vi "Parse updateConnectionState.vi"(8 "error in (no error)":errorcluster, 11 "JSON (UTF-8) String":string) -> (0 "error out":errorcluster, 2 "Telegram State":T1)   [LabVIEW 2015, in "JSON Library.lvlib"]
doc: "Created IvanLis by LabVIEW Portal\nProfile: http://labviewportal.org/memberlist.php?mode=viewprofile&u=987\neMail: IvanLisanov@gMail.com\nTelegram: https://t.me/IvanLis"
uses:
  JSON Library.lvlib
  Telegram Library/TypeDef/Telegram State.ctl
  Telegram Library/Telegram Library.lvlib
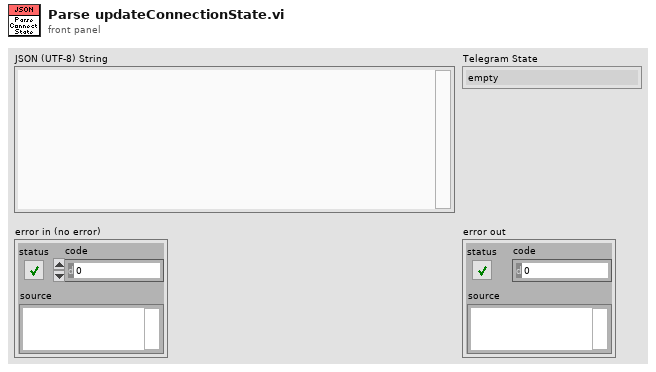
[diagram p1: front panel]
types:
  T1 = typedef "Telegram Library.lvlib/Telegram State.ctl" = enum16{"empty", "ok", "authorizationStateClosed", "authorizationStateWaitTdlibParameters", "authorizationStateWaitEncryptionKey", "authorizationStateWaitPhoneNumber", "authorizationStateWaitCode", "connectionStateWaitingForNetwork", "connectionStateConnectingToProxy", "connectionStateUpdating", "connectionStateConnecting", "connectionStateReady", "updateUser_user", "updateNewChat_chat", "updateNewMessage_Text", "updateChatLastMessage_Text", "updateDeleteMessages", "updateChatPosition", "ChatHistoryMessages_Text"}
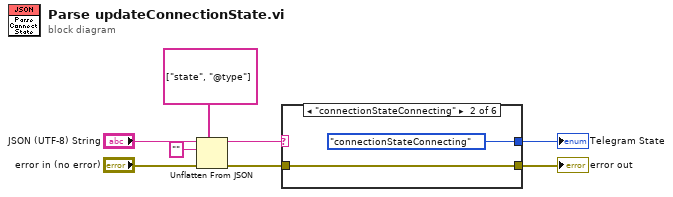
[diagram p0: block diagram]
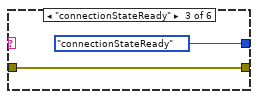
[diagram p3: hidden frame]
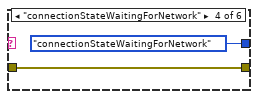
[diagram p4: hidden frame]
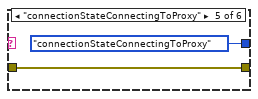
[diagram p5: hidden frame]
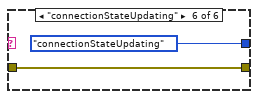
[diagram p6: hidden frame]
diagram:
  n1 = Unflatten From JSON(path=string[] ["state", "@type"], JSON string="JSON (UTF-8) String", type and defaults="", error in (no error)="error in (no error)") -> (value=w6:string, error out=w5:errorcluster)  [unwired: 3 in]
  n2 = case shown="\"connectionStateConnecting\"" w6 {
    tunnel: [_ Telegram_State."connectionStateConnecting" ("Telegram State") Telegram_State."connectionStateReady" ("Telegram State") Telegram_State."connectionStateWaitingForNetwork" ("Telegram State") Telegram_State."connectionStateConnectingToProxy" ("Telegram State") Telegram_State."connectionStateUpdating" ("Telegram State")] -> w3
    tunnel: [w9 w10 w12 w14 w16 w18] -> w4
    tunnel: w5 -> [w9 w10 w12 w14 w16 w18]
    frame Default {
    }
    frame "connectionStateConnecting" {
    }
    frame "connectionStateReady" {
    }
    frame "connectionStateWaitingForNetwork" {
    }
    frame "connectionStateConnectingToProxy" {
    }
    frame "connectionStateUpdating" {
    }
  }
  "error out" <- w4
  "Telegram State" <- w3
